vi "Init.vi"(8 "error in (no error)":errorcluster, 10 "Database":refnum<class "Database Platform.lvclass">) -> (0 "error out":errorcluster, 3 "Query Builder out":refnum<class "Query Builder.lvclass">)   [LabVIEW 2022 SP3, in "Conditum.lvlib" / "Query Builder.lvclass"]
uses:
  Query Builder.lvclass
  Database Platform/Database Platform.lvclass
  Query Builder.lvclass/Query Builder.ctl
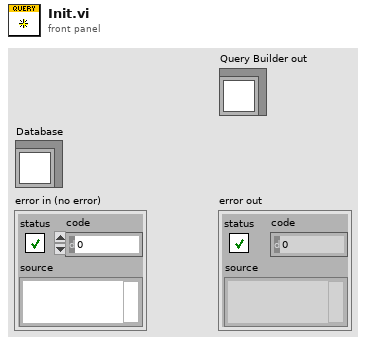
[diagram p1: front panel]
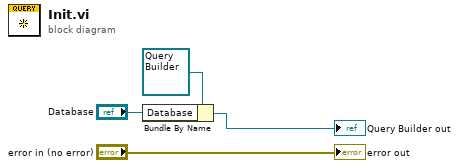
[diagram p0: block diagram]
diagram:
  n1 = Bundle By Name(cluster=refnum<class "Query Builder.lvclass"> refnum ("Query Builder in"), "Database"="Database") -> (→"Query Builder out":refnum<class "Query Builder.lvclass">)
  "error out" <- "error in (no error)"
